vi "DUT TXT BAT.vi"(8 "error in (no error)":errorcluster, 11 "command line":string="D:\\Project\\RFP_Auto\\Scripts\\Flash_once.bat") -> (0 "error out":errorcluster, 2 "Log Path":string, 3 "Result":bool)   [LabVIEW 2024]
uses:
  <vilib>/Utility/error.llb/Trim Whitespace One-Sided.vi
panel:
  out "Result":string
  out "standard output":string
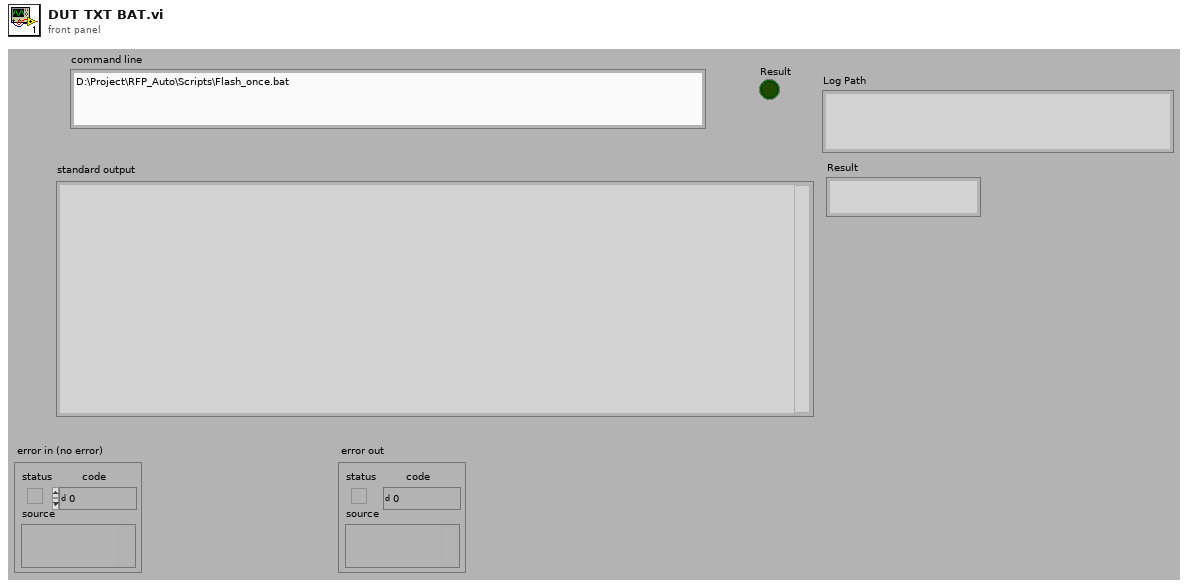
[diagram p1: front panel]
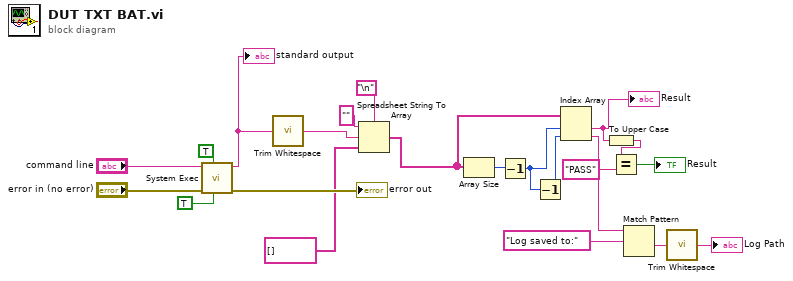
[diagram p0: block diagram]
diagram:
  n1 = call <vilib>:"System Exec.vi"("run minimized? (F)"=TRUE, "wait until completion? (T)"=TRUE, "error in (no error)"="error in (no error)", "command line"="command line") -> ("error out"=→"error out":errorcluster, "standard output"=w18:string)  [unwired: 2 in, 4 out]
  "standard output" <- w18
  n2 = call <vilib>:"Trim Whitespace.vi"("string"=w18) -> ("trimmed string"=w14:string)  [unwired: 1 in]
  n3 = Spreadsheet String To Array(delimiter (Tab)="\n", format string="", spreadsheet string=w14, array type (2D Dbl)=string[] []) -> (array=w13:string[])
  n4 = Array Size(array=w13) -> (size(s)=w12:i32)
  n5 = Decrement(x=w12) -> (x-1=w8:i32)
  n6 = Decrement(x=w8) -> (x-1=w7:i32)
  n7 = Index Array(array=w13, index #1=w8, index #2=w7) -> (element #1=w1:string, element #2=w6:string)
  "Result" <- w1
  n8 = To Upper Case(1:w1) -> (0:w2:string)
  n9 = Equal?(x=w2, y="PASS") -> (x = y?=→"Result":bool)
  n10 = Match Pattern(string=w6, regular expression="Log saved to:") -> (after substring=w4:string)  [unwired: 1 in, 3 out]
  n11 = call <vilib>:"Trim Whitespace.vi"("string"=w4) -> ("trimmed string"=→"Log Path":string)  [unwired: 1 in]
